vi "Get System Exit Message Transport.vi"(11 "Mediated Actor in":refnum<class "Mediated Actor.lvclass">) -> (2 "System Exit MT":refnum<class "Message Transport Queue.lvclass">, 3 "Mediated Actor out":refnum<class "Mediated Actor.lvclass">)   [LabVIEW 2016, in "Stream Mediator.lvlib" / "Mediated Actor.lvclass"]
uses:
  <userlib>/Composed Systems/Stream/Mediator/Classes/Mediated Actor/Mediated Actor.lvclass
  <userlib>/Composed Systems/Stream/Mediator/Classes/Message Transport Queue/Message Transport Queue.lvclass
  <userlib>/Composed Systems/Stream/Mediator/Classes/Mediated Actor/Mediated Actor.lvclass/Mediated Actor.ctl
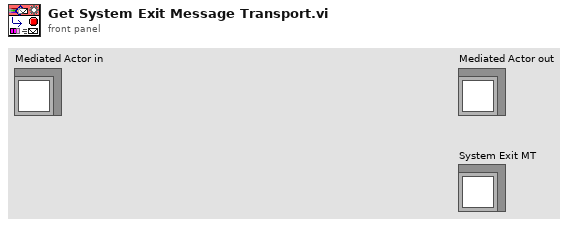
[diagram p1: front panel]
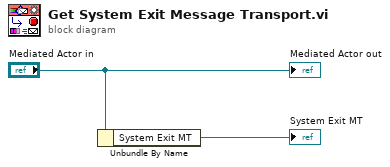
[diagram p0: block diagram]
diagram:
  n1 = Unbundle By Name("Mediated Actor in") -> ("System Exit MT"=→"System Exit MT":refnum<class "Message Transport Queue.lvclass">)
  "Mediated Actor out" <- "Mediated Actor in"
